vi "GeigerCountRate.vi"() -> ()   [LabVIEW 2014]
uses:
  <vilib>/Platform/TimedLoop/XDataNode/timing_clust.ctl
  <vilib>/Platform/TimedLoop/XDataNode/nitl_modes.ctl
  <vilib>/Platform/TimedLoop/XDataNode/wakeup.ctl
  <vilib>/Waveform/WDTFileIO.llb/ Write Waveform to File.vi
  <vilib>/platform/TimedLoop/XDataNode/XDataNode.xnode
  <vilib>/Platform/TimedLoop/XDataNode/XDNodeRunTimeDep.lvlib
panel:
  in  "Data File":path=path "C:/Users/cnee1/Desktop/week8/decay"
  out "Waveform Graph":waveform(dbl)(graph)={"t0"=timestamp(0 s since 1904-01-01), "dt"=1.0, "Y"=[23.0, 17.0, 26.0, 15.0, 18.0, 27.0, 19.0, 22.0, 32.0, 29.0, 26.0, 30.0, 23.0, 34.0, 24.0, 33.0, 32.0, 22.0, 29.0, 20.0, 35.0, 37.0, 38.0, 27.0, 27.0, 28.0, 32.0, 30.0, 17.0, 33.0, 29.0, 26.0, 23.0, 27.0, 26.0, 36.0, 30.0, 28.0, 25.0, 29.0, 35.0, 29.0, 18.0, 26.0, 36.0, 23.0, 37.0, 29.0, 22.0, 29.0, 26.0, 26.0, 31.0, 29.0, 33.0, 29.0, 25.0, 27.0, 28.0, 18.0, 23.0, 22.0, 21.0, 18.0, 24.0, 23.0, 32.0, 29.0, 27.0, 25.0, 19.0, 22.0, 20.0, 20.0, 28.0, 18.0, 17.0, 22.0, 24.0, 31.0, 23.0, 20.0, 18.0, 24.0, 24.0, 22.0, 21.0, 21.0, 21.0, 25.0, 24.0, 28.0, 28.0, 20.0, 20.0, 35.0, 20.0, 26.0, 18.0, 19.0, 14.0, 15.0, 16.0, 20.0, 21.0, 28.0, 20.0, 24.0, 21.0, 21.0, 24.0, 21.0, 15.0, 22.0, 16.0, 17.0, 17.0, 23.0, 19.0, 17.0, 19.0, 12.0, 19.0, 21.0, 22.0, 25.0, 22.0, 26.0, 24.0, 17.0, 19.0, 15.0, 23.0, 25.0, 17.0, 18.0, 15.0, 17.0, 19.0, 23.0, 13.0, 19.0, 17.0, 17.0, 29.0, 13.0, 16.0, 13.0, 15.0, 14.0, 14.0, 19.0, 31.0, 20.0, 16.0, 19.0, 21.0, 13.0, 11.0, 15.0, 21.0, 18.0, 11.0, 17.0, 11.0, 17.0, 20.0, 11.0, 26.0, 14.0, 17.0, 19.0, 21.0, 13.0, 17.0, 15.0, 16.0, 15.0, 12.0, 20.0, 17.0, 15.0, 12.0, 14.0, 22.0, 15.0, 11.0, 17.0, 16.0, 13.0, 12.0, 13.0, 21.0, 19.0, 19.0, 20.0, 12.0, 24.0, 16.0, 15.0, 22.0, 16.0, 7.0, 13.0, 13.0, 16.0, 26.0, 16.0, 21.0, 18.0, 13.0, 19.0, 15.0, 8.0, 20.0, 11.0, 18.0, 19.0, 21.0, 18.0, 17.0, 11.0, 11.0, 9.0, 12.0, 12.0, 12.0, 18.0, 12.0, 19.0, 18.0, 19.0, 12.0, 16.0, 21.0, 13.0, 13.0, 12.0, 16.0, 8.0, 16.0, 11.0, 15.0, 13.0, 19.0, 17.0, 15.0, 18.0, 18.0, 14.0, 12.0, 7.0, 10.0, 22.0, 15.0, 10.0, 15.0, 19.0, 17.0, 9.0, 11.0, 15.0, 12.0, 21.0, 13.0, 16.0, 14.0, 13.0, 10.0, 11.0, 19.0, 9.0, 12.0, 17.0, 20.0, 7.0, 18.0, 15.0, 13.0, 12.0, 15.0, 14.0, 17.0, 13.0, 12.0, 16.0, 15.0, 22.0, 12.0, 12.0, 9.0, 18.0, 16.0, 13.0, 18.0, 15.0, 12.0, 16.0, 20.0, 11.0]}
  in  "Total Time (s)":dbl=300.0
  in  "Msmt Time (s)":dbl=1.0
  out "counts per second":dbl(knob)=11.0 scale=0.0..100.0
  in  "stop":bool
  # "Count Rate"
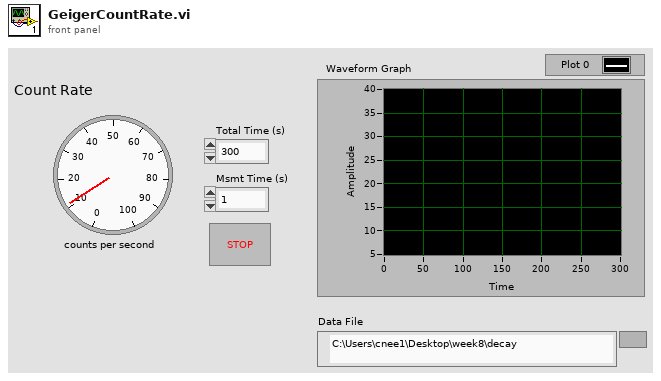
[diagram p1: front panel]
types:
  T1 = typedef "XDNodeRunTimeDep.lvlib/timing_clust.ctl" = cluster{"Expected End [f-1]":u64, "Actual End [f-1]":u64, "Finished Late? [f-1]":bool, "Expected End [i-1]":u64, "Actual End [i-1]":u64, "Finished Late? [i-1]":bool, "Expected Start [i]":u64, "Actual Start [i]":u64, "Expected Start [f]":u64, "Actual Start [f]":u64, "Source Name":string, "Structure Name":string, "Period":i64, "Deadline":i64, "Offset":i64, "Start":i64, "Priority":i32, "Timeout":i32, "Mode":T2, "Wakeup Reason":T3, "Error":errorcluster, "Source Type":string, "Secondary Source Type":string, "Global End Time":u64, "Global Start Time":u64, "Frame Duration":u64, "Iteration Duration":u64, "Assigned CPU":i32, "I/O Scan Engine Mode":u32}
  T2 = typedef "XDNodeRunTimeDep.lvlib/nitl_modes.ctl" = enum32{"No Change", "Process missed periods, maintain original phase", "Discard missed periods, maintain original phase", "Process missed periods, ignore original phase", "Discard missed periods, ignore original phase"}
  T3 = typedef "XDNodeRunTimeDep.lvlib/wakeup.ctl" = enum32{"Normal", "Aborted", "Asynchronous wakeup", "Timing source error", "Timed loop error", "Timeout"}
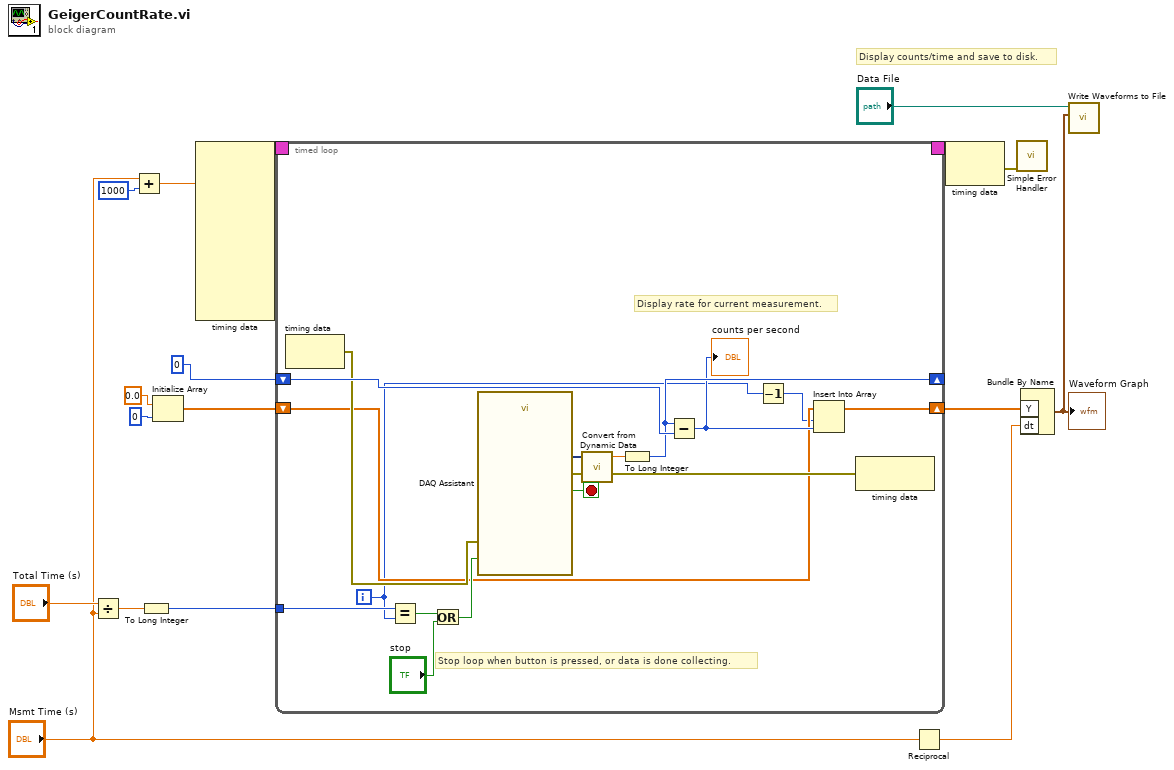
[diagram p0: block diagram]
diagram:
  # "Display counts/time and save to disk."
  n1 = Divide(x="Total Time (s)", y="Msmt Time (s)") -> (x/y=w3:dbl)
  n2 = Add(x="Msmt Time (s)", y=1000) -> (x+y=w12:dbl)
  n3 = To Long Integer(number=w3) -> (32bit integer=w8:i32)
  n4 = Initialize Array(0.0 ("element"), 0 ("dimension size")) -> (w10:dbl[])
  n5 = node-c288(w12) -> (w17:T1)  [unwired: 9 in]
  n6 = timed-loop {
    timing: w17 -> [_]
    timing-out: [_] -> w16
    shift-right: [w27] -> _
    shift-left: 0 -> [w32]
    tunnel: w8 -> [w26]
    shift-right: [w19] -> w5
    shift-left: w10 -> [w21]
    i -> [w20]
    stop <- w31 stop-if-true
    # "Stop loop when button is pressed, or data is done collecting."
    # "Display rate for current measurement."
    n7 = node-c288() -> (w28:errorcluster)  [unwired: 1 in]
    n8 = Equal?(x=w26, y=w20) -> (x = y?=w24:bool)
    n9 = Or(x=w24, y="stop") -> (x .or. y?=w23:bool)
    n10 = call "DAQ Assistant"("error in"=w28, "stop (F)"=w23) -> ("data"=w33:dynamicdata, "stopped"=w31:bool, "error out"=w29:errorcluster)  [unwired: 14 in, 1 out]
    n11 = call "Convert from Dynamic Data"("Dynamic Data Type"=w33) -> ("Scalar"=w30:dbl)  [unwired: 3 in]
    n12 = To Long Integer(number=w30) -> (32bit integer=w27:i32)
    n13 = Subtract(x=w27, y=w32) -> (x-y=w22:i32)
    "counts per second" <- w22
    n14 = Decrement(x=w20) -> (x-1=w18:i32)
    n15 = Insert Into Array(array=w21, index=w18, new element=w22) -> (w19:dbl[])
    n16 = node-c288(w29) -> ()  [unwired: 1 out]
  }
  n17 = Reciprocal(x="Msmt Time (s)") -> (1/x=w4:dbl)
  n18 = node-c288(w16) -> (w14:errorcluster)
  n19 = call <vilib>:"Simple Error Handler.vi"("error in (no error)"=w14) -> ()  [unwired: 4 in, 5 out]
  n20 = Bundle By Name("Y"=w5, "dt"=w4) -> (w2:waveform(dbl))  [unwired: 1 in]
  "Waveform Graph" <- w2
  n21 = call-poly <vilib>:"Write Waveforms to File.vi"("waveform"=w2, "file path (dialog if empty)"="Data File") -> ()  [unwired: 8 in, 2 out]
